vi "Initialise HIL Mode.vi"(8 "error in":errorcluster, 9 "Analog In Data Size":T1, 10 "Samples to Read":i32, 11 "configuration file path":path) -> (0 "error out":errorcluster, 1 "Ready":bool)   [LabVIEW 2017, in "DTACQ - Network Enabled Device Driver.lvlib"]
doc: "Prepare the Dtacq device for hardare-in-the-loop mode;\n-Loads INI file\n-Sets the data size (16 or 32 bit data)\n-Clears any unfinished shots\n-Stores the INI settings, samples to read and data size as functional global variables"
uses:
  DTACQ - Network Enabled Device Driver.lvlib
  Communications/Typedefs/Data Size--Enum.ctl
  Driver Global Settings--Typedef.ctl
  Communications/Typedefs/DTACQ Connection Data--Cluster.ctl
  FGV Operaions--Enum.ctl
  Communications/Communications Library.lvlib
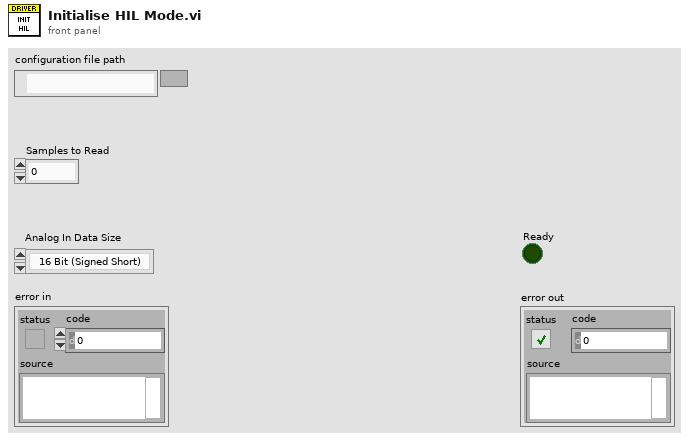
[diagram p1: front panel]
types:
  T1 = typedef "Communications Library.lvlib/Data Size--Enum.ctl" = enum16{"16 Bit (Signed Short)", "32 Bit (Signed Long)"}
  T2 = typedef "DTACQ - Network Enabled Device Driver.lvlib/FGV Operaions--Enum.ctl" = enum16{"Get Driver Settings", "Set Driver Settings", "Search Variable Names", "Close Connections", "Open Connections", "Get Variable References", "Set Variable References", "Clear"}
  T3 = typedef "DTACQ - Network Enabled Device Driver.lvlib/Driver Global Settings--Typedef.ctl" = cluster{"Waveform Length":i32, "Data Size":T1, "DTACQ Connection Data":T4}
  T4 = typedef "Communications Library.lvlib/DTACQ Connection Data--Cluster.ctl" = cluster{"Description":string, "Address":string, "Port":u16, "timeout (ms)":i32, "Termination Character":string, "TCP Connection Reference":refnum<k5>, "Open Connection":bool}
  T5 = typedef "Communications Library.lvlib/DTACQ Module Carrier Configuration--Cluster.ctl" = cluster{"Name":string, "IP":string, "Control Port":i32, "Timeout (ms)":i32, "Continuous Capture Port (Multiplexed)":i32, "Start HIL Shot Port":i32, "AWG Upload Port (Multiplexed)":i32, "Download Captured Data Port (Multiplexed)":i32, "Module Slots":i32, "Module Configurations":T6[]}
  T6 = typedef "Communications Library.lvlib/DTACQ Module Configuration--Cluster.ctl" = cluster{"Name":string, "Position":string, "Module Type":T7, "Control Port":i32, "Timeout (ms)":i32, "Channels":i32}
  T7 = typedef "Communications Library.lvlib/DTACQ Device Type--Enum.ctl" = enum16{"Carrier", "Analog In Module", "Analog Out Module", "Generic Module"}
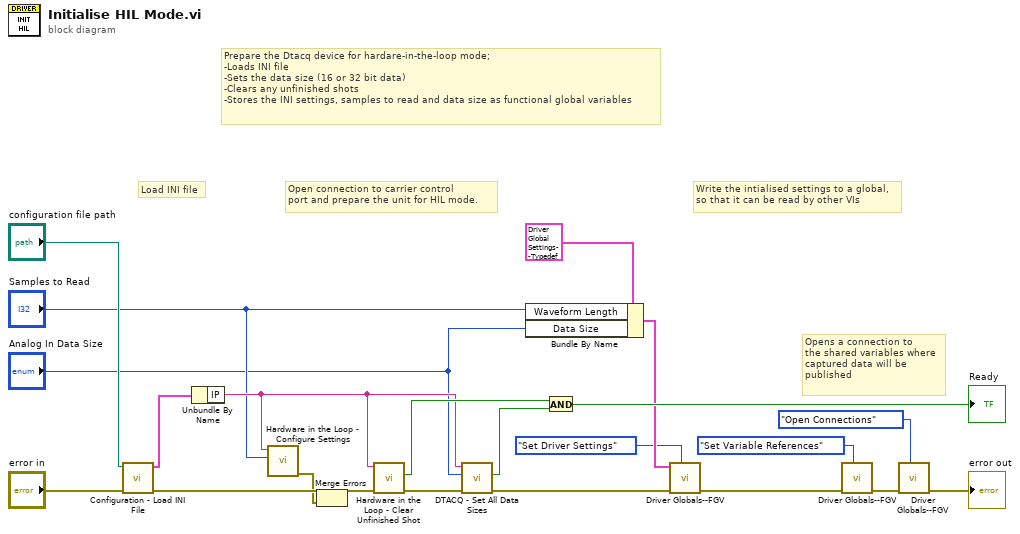
[diagram p0: block diagram]
diagram:
  # "Opens a connection to \nthe shared variables where\ncaptured data will be \npublished"
  # "Prepare the Dtacq device for hardare-in-the-loop mode;\n-Loads INI file\n-Sets the data size (16 or 32 bit data)\n-Clears any unfinished shots\n-Stores the INI settings, samples to read and data size as functional global variables"
  # "Open connection to carrier control\nport and prepare the unit for HIL mode."
  # "Load INI file"
  # "Write the intialised settings to a global,\nso that it can be read by other VIs"
  n1 = call "Configuration - Load INI File.vi"("error in"="error in", "configuration file path"="configuration file path") -> ("error out"=w15:errorcluster, "Carrier Configuration Out"=w17:T5)  [unwired: 8 in]
  n2 = Unbundle By Name(w17) -> ("IP"=w16:string)
  n3 = call "Hardware in the Loop - Configure Settings.vi"("Samples to Read"="Samples to Read", "Address"=w16) -> ("error out"=w14:errorcluster)  [unwired: 9 in]
  n4 = Merge Errors(w15, w14) -> (w13:errorcluster)
  n5 = call "Hardware in the Loop - Clear Unfinished Shot.vi"("error in"=w13, "Address"=w16) -> ("error out"=w22:errorcluster, "Ready"=w20:bool)  [unwired: 8 in]
  n6 = call "DTACQ - Set All Data Sizes.vi"("error in"=w22, "Analog In Data Size"="Analog In Data Size", "Address"=w16) -> ("error out"=w3:errorcluster, "Acknowledged"=w21:bool)  [unwired: 7 in]
  n7 = Bundle By Name(cluster=T3 {"Waveform Length"=0, "Data Size"=enum."16 Bit (Signed Short)", "DTACQ Connection Data"={"Description"="", "Address"="", "Port"=0, "timeout (ms)"=5000, "Termination Character"="\n", "TCP Connection Reference"=refnum, "Open Connection"=FALSE}} ("Driver Settings In"), "Waveform Length"="Samples to Read", "Data Size"="Analog In Data Size") -> (w9:T3)
  n8 = And(x=w20, y=w21) -> (x .and. y?=→"Ready":bool)
  n9 = call "Driver Globals--FGV.vi"(7:FGV_Operaions--Enum."Set Driver Settings", "error in"=w3, "Driver Settings In"=w9) -> ("error out"=w2:errorcluster)  [unwired: 5 in, 3 out]
  n10 = call "Driver Globals--FGV.vi"(7:FGV_Operaions--Enum."Set Variable References", "error in"=w2) -> ("error out"=w5:errorcluster)  [unwired: 6 in, 3 out]
  n11 = call "Driver Globals--FGV.vi"(7:FGV_Operaions--Enum."Open Connections", "error in"=w5) -> ("error out"=→"error out":errorcluster)  [unwired: 6 in, 3 out]
